vi "TrigTest.vi"() -> (0 "error out":errorcluster, 2 "Boolean":bool, 3 "Waveform Graph":dynamicdata(graph))   [LabVIEW 2012]
panel:
  in  "stop (F)":bool
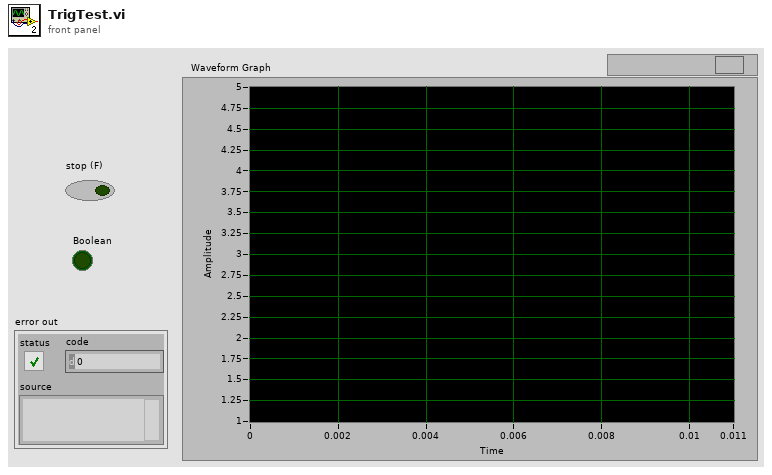
[diagram p1: front panel]
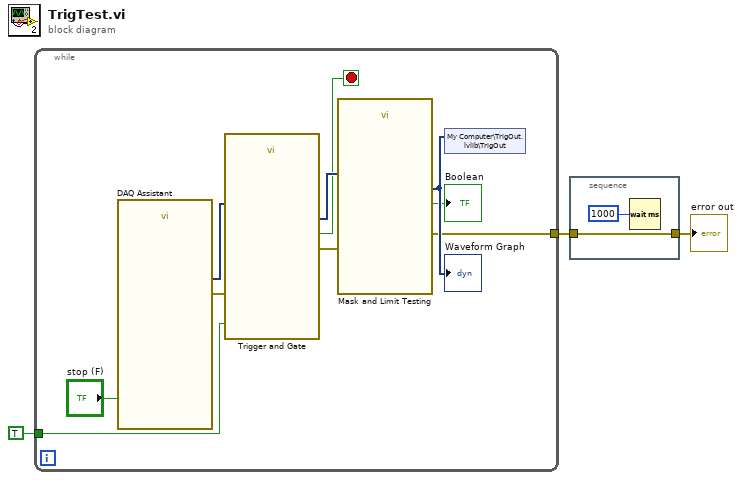
[diagram p0: block diagram]
diagram:
  n1 = while {
    tunnel: [w7] -> w3
    tunnel: TRUE ("Reset") -> [w4]
    stop <- w5 stop-if-true
    n2 = call "DAQ Assistant"("stop (F)"="stop (F)") -> ("data"=w12:dynamicdata, "error out"=w9:errorcluster)  [unwired: 15 in, 2 out]
    n3 = call "Trigger and Gate"("error in (no error)"=w9, "Reset"=w4, "Signals"=w12) -> ("error out"=w8:errorcluster, "Triggered Signals"=w11:dynamicdata, "Data Available"=w5:bool)  [unwired: 5 in, 1 out]
    n4 = call "Mask and Limit Testing"("error in"=w8, "Signals"=w11) -> ("error out"=w7:errorcluster, "Passed"=→"Boolean":bool, "Tested Signals"=w10:dynamicdata)  [unwired: 6 in, 1 out]
    "Waveform Graph" <- w10
    n5 = shared-variable "My Computer\\TrigOut.lvlib\\TrigOut"(w10) -> ()  [unwired: 1 in, 1 out]
  }
  n6 = stacked-sequence {
    tunnel: w3 -> [w14]
    tunnel: [w14] -> w2
    frame #0 {
      n7 = Wait (ms)(milliseconds to wait=u32 1000) -> ()  [unwired: 1 out]
    }
  }
  "error out" <- w2
